vi "Configure Pulser Range.vi"(6 "Voltage Range (10V)":i32(ring)=1 items=["5", "10"], 7 "Current Range (10A)":i32(ring)=2 items=["1", "5", "10", "0.250000"], 8 "error in (no error)":errorcluster, 10 "Source Measure Unit Channel (0: Channel A)":i32(ring) items=["Channel A", "Channel B"], 11 "VISA resource name":refnum<visa-resource-name>) -> (0 "error out":errorcluster, 3 "VISA resource name out":refnum<visa-resource-name>)   [LabVIEW 2015, in "Keithley 2600 Series.lvlib"]
doc: "Sets source and measure ranges when the Pulser is enabled"
uses:
  Keithley 2600 Series.lvlib
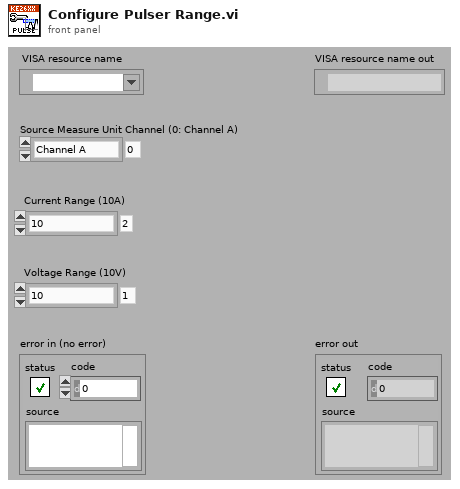
[diagram p1: front panel]
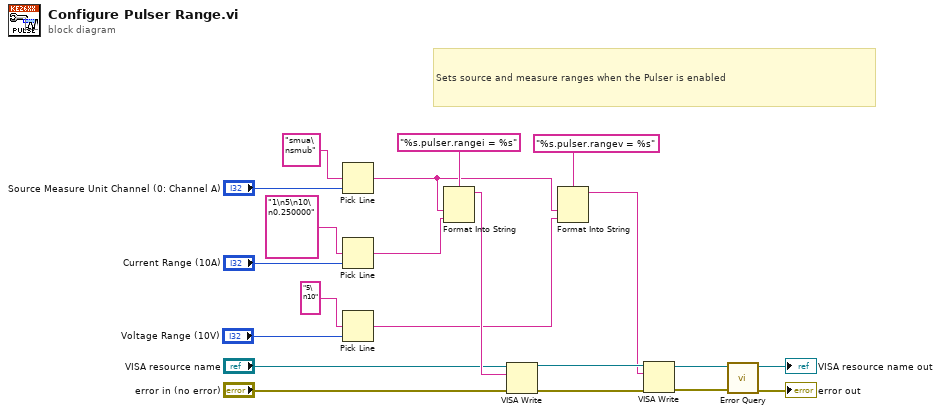
[diagram p0: block diagram]
diagram:
  # "Sets source and measure ranges when the Pulser is enabled"
  n1 = Pick Line(multi-line string="smua\nsmub", line index="Source Measure Unit Channel (0: Channel A)") -> (output string=w14:string)  [unwired: 1 in]
  n2 = Pick Line(multi-line string="1\n5\n10\n0.250000", line index="Current Range (10A)") -> (output string=w4:string)  [unwired: 1 in]
  n3 = Pick Line(multi-line string="5\n10", line index="Voltage Range (10V)") -> (output string=w1:string)  [unwired: 1 in]
  n4 = Format Into String(format string="%s.pulser.rangei = %s", w14, w4) -> (resulting string=w18:string)  [unwired: 2 in, 1 out]
  n5 = VISA Write(VISA resource name="VISA resource name", write buffer=w18, error in (no error)="error in (no error)") -> (VISA resource name out=w10:refnum<visa-resource-name>, error out=w13:errorcluster)  [unwired: 1 out]
  n6 = Format Into String(format string="%s.pulser.rangev = %s", w14, w1) -> (resulting string=w9:string)  [unwired: 2 in, 1 out]
  n7 = VISA Write(VISA resource name=w10, write buffer=w9, error in (no error)=w13) -> (VISA resource name out=w11:refnum<visa-resource-name>, error out=w12:errorcluster)  [unwired: 1 out]
  n8 = call "Error Query.vi"("error in (no error)"=w12, "VISA resource name"=w11) -> ("error out"=→"error out":errorcluster, "VISA resource name out"=→"VISA resource name out":refnum<visa-resource-name>)  [unwired: 6 in, 2 out]
